vi "Signal Playback.vi"(6 "Sampling info":cluster{"Fs":dbl, "#s":dbl}, 8 "error in (no error)":errorcluster, 9 "Queue in":refnum<queue>, 10 "Event in":refnum<user-event>) -> (0 "error out":errorcluster)   [LabVIEW 2019]
uses:
  Type Definitions/Machine States/Signal Playback State.ctl
  Type Definitions/DataInOut.ctl
  <vilib>/sound2/lvsound2.llb/Sampling Mode.ctl
  <vilib>/sound2/lvsound2.llb/Sound Data Format.ctl
  <vilib>/sound2/lvsound2.llb/Sound Output Set Volume (Single).vi
  <vilib>/sound2/lvsound2.llb/Sound Output Write (DBL Single).vi
panel:
  out "State":T1
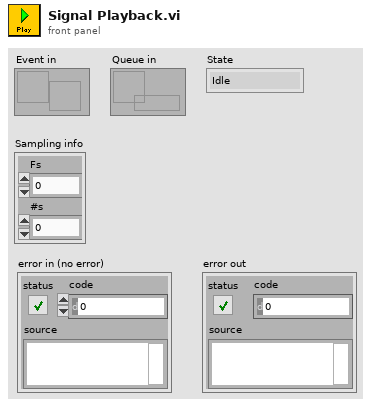
[diagram p1: front panel]
types:
  T1 = typedef "Signal Playback State.ctl" = enum16{"Idle", "Initialization", "Playing", "End"}
  T2 = typedef "DataInOut.ctl" = enum16{"Write", "Read"}
  T3 = typedef "Sound Data Format.ctl" = cluster{"sample rate (S/s)":dbl, "number of channels":i32, "bits per sample":i32}
  T4 = typedef "Sampling Mode.ctl" = i32
  T5 = typedef "Sound Output Task ID.ctl" = u32
  T6 = typedef "UI.ctl" = cluster{"Oscillator":T7, "VCA":T9, "Lowpass filter":T10, "Tremolo":T11, "Play sound":bool, "Stop Application":bool}
  T7 = typedef "UIOscillatorParam.ctl" = cluster{"Waveform Type":u16, "Pulse Width":dbl, "Sub oscillator":T8, "Frequency":dbl}
  T8 = typedef "Sub Oscillalator Type.ctl" = enum16{"Off", "One Octave", "Two Octaves"}
  T9 = typedef "UIADSRParam.ctl" = cluster{"A":i32, "D":i32, "S":i32, "R":i32, "Volume":dbl}
  T10 = typedef "UILowpassParam.ctl" = cluster{"On / Off":bool, "Cutoff":dbl}
  T11 = typedef "UITremolo.ctl" = cluster{"Rate":dbl, "Frequency":dbl, " on/off ":bool}
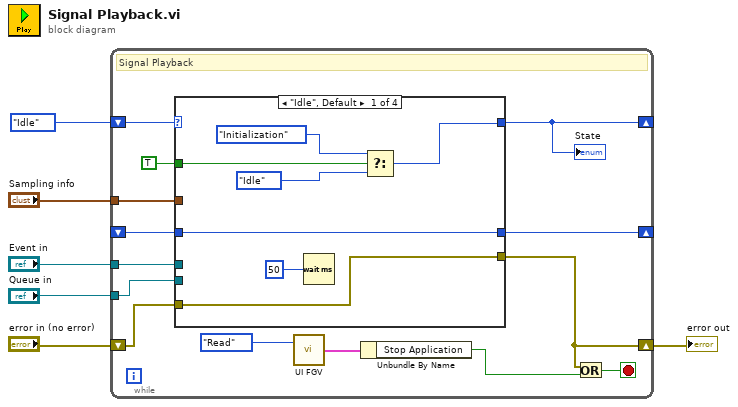
[diagram p0: block diagram]
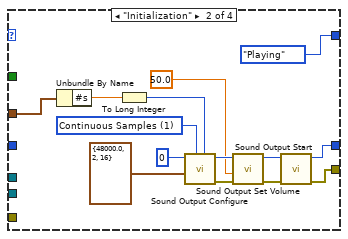
[diagram p2: hidden frame]
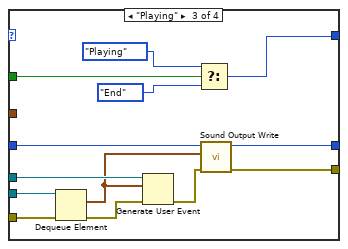
[diagram p3: hidden frame]
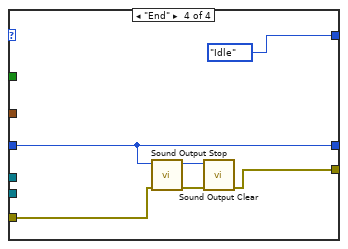
[diagram p4: hidden frame]
diagram:
  n1 = while {
    shift-right: [w16] -> w3
    shift-left: "error in (no error)" -> [w19]
    shift-right: [w11] -> _
    shift-left: Signal_Playback_State."Idle" -> [w20]
    shift-right: [w15] -> _
    shift-left: _ -> [w18]
    tunnel: "Queue in" -> [w14]
    tunnel: "Sampling info" -> [w13]
    tunnel: "Event in" -> [w12]
    stop <- w17 stop-if-true
    # "Signal Playback"
    n2 = case shown="\"Idle\", Default" w20 {
      tunnel: [w27 w36 w42 w56] -> w16
      tunnel: w19 -> [w27 _ w54 w57]
      tunnel: TRUE ("Play") -> [w22 _ w50 _]
      tunnel: [w21 Signal_Playback_State."Playing" ("f") w46 Signal_Playback_State."Idle" ("f")] -> w11
      tunnel: w18 -> [w23 _ w44 w58]
      tunnel: w14 -> [_ _ w51 _]
      tunnel: [w23 w35 w45 w58] -> w15
      tunnel: w13 -> [_ w34 _ _]
      tunnel: w12 -> [_ _ w49 _]
      frame "Idle", Default {
        n3 = Wait (ms)(milliseconds to wait=u32 50) -> ()  [unwired: 1 out]
        n4 = Select(t=Signal_Playback_State."Initialization", s=w22, f=Signal_Playback_State."Idle") -> (s? t:f=w21:T1)
      }
      frame "Initialization" {
        w37 = T4 1 items=["Finite Samples", "Continuous Samples"] ("sample mode")
        n5 = Unbundle By Name(w34) -> ("#s"=w32:dbl)
        n6 = To Long Integer(number=w32) -> (32bit integer=w33:i32)
        n7 = call <vilib>:"Sound Output Configure.vi"("number of samples/ch"=w33, "sample mode"=w37, "sound format"=T3 {"sample rate (S/s)"=48000.0, "number of channels"=2, "bits per sample"=16}, "device ID"=u32 0) -> ("error out"=w38:errorcluster, "task ID"=w39:T5)  [unwired: 6 in]
        n8 = call-poly <vilib>:"Sound Output Set Volume.vi"("error in (no error)"=w38, "volume"=50.0, "task ID"=w39) -> ("error out"=w41:errorcluster, "task ID out"=w40:T5)  [unwired: 7 in]
        n9 = call <vilib>:"Sound Output Start.vi"("error in (no error)"=w41, "task ID"=w40) -> ("error out"=w36:errorcluster, "task ID out"=w35:T5)  [unwired: 8 in]
      }
      frame "Playing" {
        n10 = Dequeue Element(queue=w51, error in (no error)=w54) -> (element=w47:waveform(dbl), error out=w48:errorcluster)  [unwired: 1 in, 2 out]
        n11 = Generate User Event(user event=w49, event data cluster=w47, error in=w48) -> (error out=w43:errorcluster)  [unwired: 1 in, 1 out]
        n12 = Select(t=Signal_Playback_State."Playing", s=w50, f=Signal_Playback_State."End") -> (s? t:f=w46:T1)
        n13 = call-poly <vilib>:"Sound Output Write.vi"("error in (no error)"=w43, "data"=w47, "task ID"=w44) -> ("error out"=w42:errorcluster, "task ID out"=w45:T5)  [unwired: 7 in]
      }
      frame "End" {
        n14 = call <vilib>:"Sound Output Stop.vi"("error in (no error)"=w57, "task ID"=w58) -> ("error out"=w59:errorcluster, "task ID out"=w60:T5)  [unwired: 8 in]
        n15 = call <vilib>:"Sound Output Clear.vi"("error in (no error)"=w59, "task ID"=w60) -> ("error out"=w56:errorcluster)  [unwired: 9 in]
      }
    }
    "State" <- w11
    n16 = call "UI FGV.vi"("Mode"=DataInOut."Read") -> ("Data out"=w8:T6)  [unwired: 1 in]
    n17 = Unbundle By Name(w8) -> ("Stop Application"=w7:bool)
    n18 = Or(x=w16, y=w7) -> (x .or. y?=w17:bool)
  }
  "error out" <- w3
